vi "Turret_Execute.vi"() -> ()   [LabVIEW 2020]
uses:
  Turret_States.ctl
  <vilib>/Rock Robotics/WPI/ThirdParty/Phoenix-LabVIEW/Motor Controller/Controls/CTRE_Phoenix_MotorControl_ControlMode.ctl
  Globals/Turret_Globals.vi
  Globals/Sensor_Values.vi
  Globals/Calibration_And_Constant_Globals.vi
panel:
  in  "max offset":dbl=2.0 format="%#_13g"
  in  "Int Error Window":dbl=2.0
  out "Controller Summary":T1(graph)
  out "goal":dbl=2.0
  in  "goal_from_center_of_target":dbl=8.0
  out "turret error":dbl
  in  "acceptable_turret_error(deg)":dbl=3.0
  in  "Disable_Limit_Safeties":bool
  out "Waveform Chart":cluster{"Goal Wheel Position":dbl, dbl}(graph)
  in  "Kd Aim":dbl
  in  "Ki Aim":dbl=0.03
  in  "upper_limit(degrees)":dbl=180.0
  in  "lower_limit(degrees)":dbl=-180.0
  out "Turret_Spin_Speed":dbl
  in  "Kp Aim":dbl=0.03
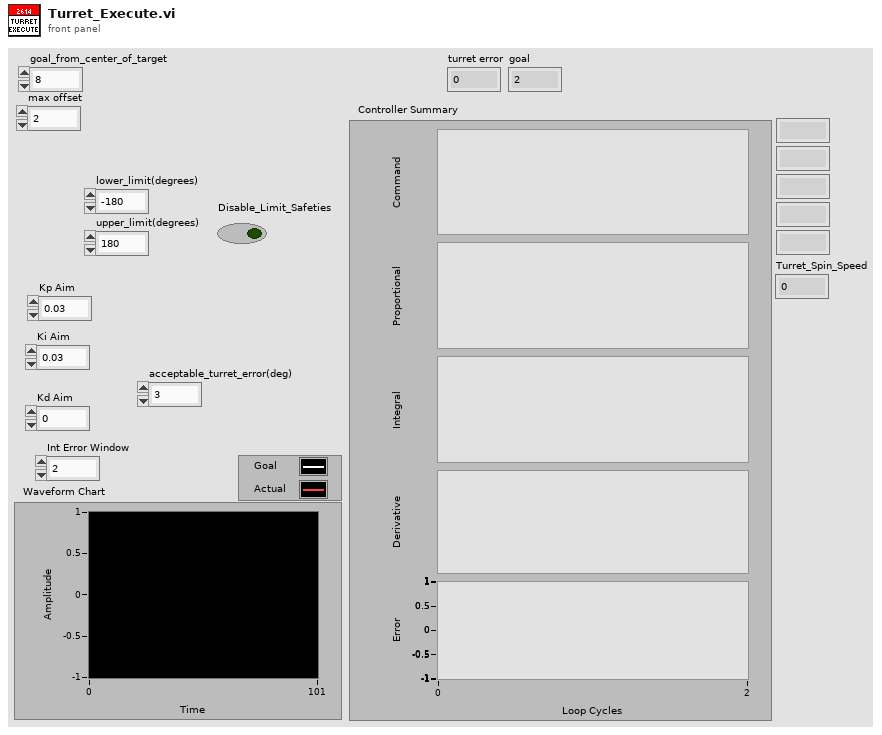
[diagram p1: front panel]
types:
  T1 = cluster{"Command":dbl, "Proportional":dbl, "Integral":dbl, "Derivative":dbl, "Goal":dbl}
  T2 = typedef "Turret_States.ctl" = enum16{"Manual_Percent_Voltage", "Target_With_Limelight", "Command_TurnToPosition", "Command_Auto_Target", "GoToZero", "No-Op", "Test_Position_Control", "Position_Control"}
  T3 = cluster{"Kp":dbl, "Ki":dbl, "Kd":dbl, "N-Diff":i32, "N-Int":i32, "Int Error Window":dbl, "Max Ouput":dbl, "Min Output":dbl}
  T4 = typedef "Turret_Cluster.ctl" = cluster{"Turret_Control_State":T2, "Manual_Speed":dbl, "Step":i32, "Parameter_1":dbl, "Parameter_2":dbl, "Parameter_3":dbl, "Auto_Notifier":refnum<notifier>, "Goal_Angle":dbl, "Camera_Goal_X":dbl}
  T5 = typedef "CTRE_Phoenix_MotorControl_ControlMode.ctl" = u16
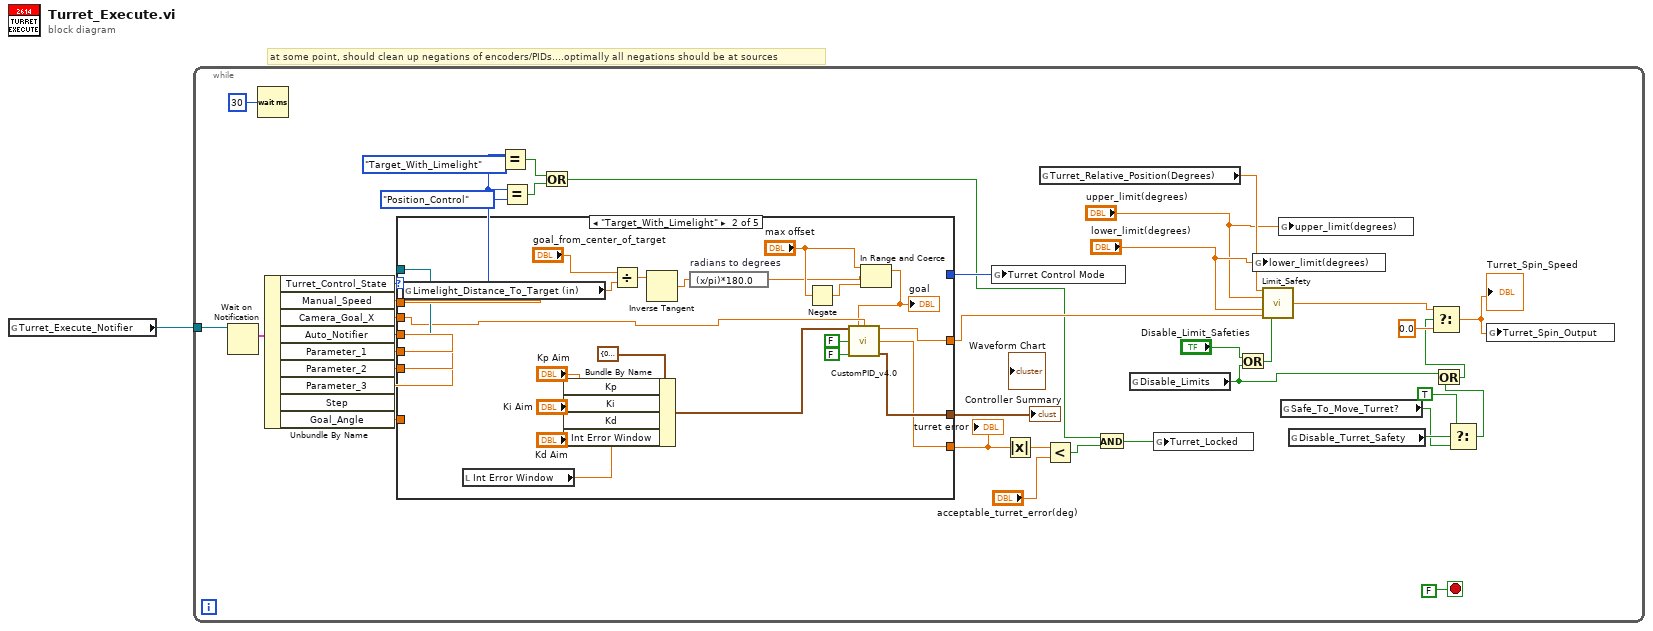
[diagram p0: block diagram]
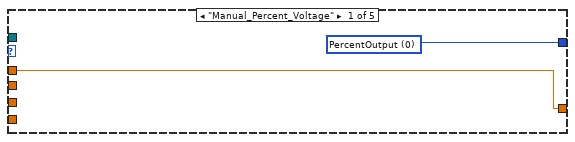
[diagram p2: hidden frame]
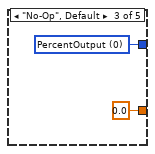
[diagram p3: hidden frame]
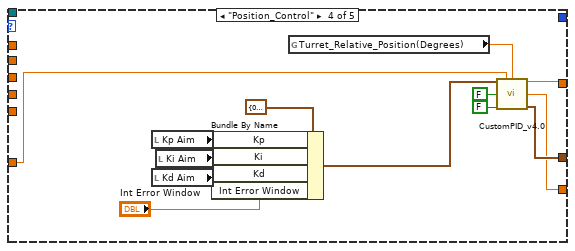
[diagram p4: hidden frame]
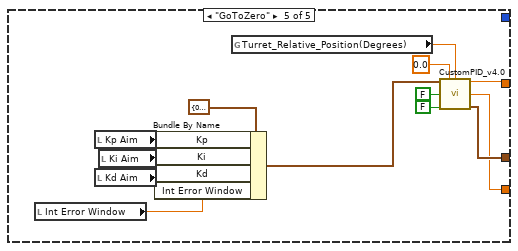
[diagram p5: hidden frame]
diagram:
  # "at some point, should clean up negations of encoders/PIDs....optimally all negations should be at sources"
  n1 = global read "Turret_Globals.vi" "Turret_Execute_Notifier"() -> (w1:refnum<notifier>)
  n2 = while {
    tunnel: w1 -> [w39]
    stop <- FALSE stop-if-true
    n3 = Wait on Notification(notifier=w39) -> (notification=w38:T4)  [unwired: 3 in, 3 out]
    n4 = Wait (ms)(milliseconds to wait=u32 30) -> ()  [unwired: 1 out]
    n5 = Unbundle By Name(w38) -> ("Turret_Control_State"=w8:T2, "Manual_Speed"=w37:dbl, "Camera_Goal_X"=w28:dbl, "Auto_Notifier"=w32:refnum<notifier>, "Parameter_1"=w35:dbl, "Parameter_2"=w34:dbl, "Parameter_3"=w33:dbl, "Goal_Angle"=w26:dbl)  [unwired: 1 out]
    n6 = case shown="\"Target_With_Limelight\"" w8 {
      tunnel: w37 -> [w42 _ _ _ _]
      tunnel: [w42 w48 0.0 ("Command") w67 w81] -> w30
      tunnel: w35 -> [_ _ _ _ _]
      tunnel: w34 -> [_ _ _ _ _]
      tunnel: w33 -> [_ _ _ _ _]
      tunnel: w32 -> [_ _ _ _ _]
      tunnel: [w41 _ w64 _ _] -> w29
      tunnel: w28 -> [_ w51 _ _ _]
      tunnel: w26 -> [_ _ _ w69 _]
      tunnel: [_ w49 _ w66 w80] -> w25
      tunnel: [_ w50 _ w68 w82] -> w2
      frame "Manual_Percent_Voltage" {
        w41 = T5 0 items=["PercentOutput"=0, "Position"=1, "Velocity"=2, "Current"=3, "Follower"=5, "MotionProfile"=6, "MotionMagic"=7, "MotionProfileArc"=10, "Disabled"=15] ("Control Mode")
      }
      frame "Target_With_Limelight" {
        n7 = global read "Sensor_Values.vi" "Limelight_Distance_To_Target (in)"() -> (w62:dbl)
        n8 = local read "Int Error Window"() -> (w47:dbl)
        n9 = Bundle By Name(cluster=T3 {"Kp"=0.1, "Ki"=0.1, "Kd"=0.1, "N-Diff"=10, "N-Int"=20, "Int Error Window"=0.5, "Max Ouput"=1.0, "Min Output"=-1.0} ("PID Tuning Parameters"), "Kp"="Kp Aim", "Ki"="Ki Aim", "Kd"="Kd Aim", "Int Error Window"=w47) -> (w58:T3)
        n10 = Divide(x="goal_from_center_of_target", y=w62) -> (x/y=w61:dbl)
        n11 = Inverse Tangent(1:w61) -> (0:w60:dbl)
        n12 = expression code="(x/pi)*180.0" "radians to degrees"(w60) -> (w44:dbl)
        n13 = Negate(x="max offset") -> (-x=w45:dbl)
        n14 = In Range and Coerce(upper limit="max offset", x=w44, lower limit=w45) -> (coerced(x)=w43:dbl)  [unwired: 1 out]
        "goal" <- w43
        n15 = call "CustomPID_v4.0.vi"("PID Tuning Parameters"=w58, "Goal"=w43, "Process Variable"=w51, "Reset on Goal Change ?"=FALSE, "Use Custom Error Calculation ?"=FALSE) -> ("Command"=w48:dbl, "Current Error"=w49:dbl, "Controller Summary"=w50:T1)  [unwired: 7 in, 1 out]
      }
      frame "No-Op", Default {
        w64 = T5 0 items=["PercentOutput"=0, "Position"=1, "Velocity"=2, "Current"=3, "Follower"=5, "MotionProfile"=6, "MotionMagic"=7, "MotionProfileArc"=10, "Disabled"=15] ("Control Mode")
      }
      frame "Position_Control" {
        n16 = local read "Kp Aim"() -> (w73:dbl)
        n17 = local read "Kd Aim"() -> (w71:dbl)
        n18 = local read "Ki Aim"() -> (w72:dbl)
        n19 = Bundle By Name(cluster=T3 {"Kp"=0.1, "Ki"=0.1, "Kd"=0.1, "N-Diff"=10, "N-Int"=20, "Int Error Window"=0.5, "Max Ouput"=1.0, "Min Output"=-1.0} ("PID Tuning Parameters"), "Kp"=w73, "Ki"=w72, "Kd"=w71, "Int Error Window"="Int Error Window") -> (w76:T3)
        n20 = global read "Sensor_Values.vi" "Turret_Relative_Position(Degrees)"() -> (w70:dbl)
        n21 = call "CustomPID_v4.0.vi"("PID Tuning Parameters"=w76, "Goal"=w69, "Process Variable"=w70, "Reset on Goal Change ?"=FALSE, "Use Custom Error Calculation ?"=FALSE) -> ("Command"=w67:dbl, "Current Error"=w66:dbl, "Controller Summary"=w68:T1)  [unwired: 7 in, 1 out]
      }
      frame "GoToZero" {
        n22 = local read "Int Error Window"() -> (w78:dbl)
        n23 = local read "Kp Aim"() -> (w86:dbl)
        n24 = local read "Kd Aim"() -> (w84:dbl)
        n25 = local read "Ki Aim"() -> (w85:dbl)
        n26 = Bundle By Name(cluster=T3 {"Kp"=0.1, "Ki"=0.1, "Kd"=0.1, "N-Diff"=10, "N-Int"=20, "Int Error Window"=0.5, "Max Ouput"=1.0, "Min Output"=-1.0} ("PID Tuning Parameters"), "Kp"=w86, "Ki"=w85, "Kd"=w84, "Int Error Window"=w78) -> (w89:T3)
        n27 = global read "Sensor_Values.vi" "Turret_Relative_Position(Degrees)"() -> (w83:dbl)
        n28 = call "CustomPID_v4.0.vi"("PID Tuning Parameters"=w89, "Goal"=0.0, "Process Variable"=w83, "Reset on Goal Change ?"=FALSE, "Use Custom Error Calculation ?"=FALSE) -> ("Command"=w81:dbl, "Current Error"=w80:dbl, "Controller Summary"=w82:T1)  [unwired: 7 in, 1 out]
      }
    }
    "turret error" <- w25
    "Controller Summary" <- w2
    n29 = Equal?(x=w8, y=Turret_States."Target_With_Limelight") -> (x = y?=w6:bool)
    n30 = Equal?(x=w8, y=Turret_States."Position_Control") -> (x = y?=w7:bool)
    n31 = Or(x=w6, y=w7) -> (x .or. y?=w5:bool)
    n32 = global write "Turret_Globals.vi" "Turret Control Mode"(w29) -> ()
    n33 = Absolute Value(x=w25) -> (abs(x)=w24:dbl)
    n34 = global read "Sensor_Values.vi" "Turret_Relative_Position(Degrees)"() -> (w27:dbl)
    n35 = Less?(x=w24, y="acceptable_turret_error(deg)") -> (x < y?=w22:bool)
    n36 = And(x=w5, y=w22) -> (x .and. y?=w21:bool)
    n37 = global read "Calibration_And_Constant_Globals.vi" "Disable_Limits"() -> (w19:bool)
    n38 = global write "Turret_Globals.vi" "Turret_Locked"(w21) -> ()
    n39 = Or(x="Disable_Limit_Safeties", y=w19) -> (x .or. y?=w18:bool)
    n40 = global write "Turret_Globals.vi" "lower_limit(degrees)"("lower_limit(degrees)") -> ()
    n41 = call "Limit_Safety.vi"("Sensor_Value"=w27, "Upper_Limit"="upper_limit(degrees)", "Lower_Limit"="lower_limit(degrees)", "Outer_Arm_Pivot_Throttle"=w30, "Disable_Limit_Safeties"=w18) -> ("Corrected Output"=w17:dbl)  [unwired: 10 in]
    n42 = global write "Turret_Globals.vi" "upper_limit(degrees)"("upper_limit(degrees)") -> ()
    n43 = global read "Sensor_Values.vi" "Safe_To_Move_Turret?"() -> (w12:bool)
    n44 = global read "Turret_Globals.vi" "Disable_Turret_Safety"() -> (w13:bool)
    n45 = Select(t=TRUE, s=w13, f=w12) -> (s? t:f=w10:bool)
    n46 = Or(x=w19, y=w10) -> (x .or. y?=w14:bool)
    n47 = Select(t=w17, s=w14, f=0.0) -> (s? t:f=w15:dbl)
    "Turret_Spin_Speed" <- w15
    n48 = global write "Turret_Globals.vi" "Turret_Spin_Output"(w15) -> ()
  }
